vi "Resize Front Panel Main.vi"(0 "Left Listbox":refnum<vi>, 1 "Top Level VI":refnum<vi>, 2 "Stop":refnum<vi>, 3 "Number of Columns":i32=4, 5 "Right Listbox":refnum<vi>, 7 "Left Splitter":refnum<vi>, 9 "Right Splitter":refnum<vi>, 11 "error in (no error)":errorcluster, 12 "Left Pane Items":refnum<vi>[](array[refnum]), 13 "Mid Pane Items":refnum<vi>[](array[refnum]), 14 "Right Pane Items":refnum<vi>[](array[refnum])) -> (15 "error out":errorcluster)   [LabVIEW 2013]
uses:
  <vilib>/Utility/miscctls.llb/LVRectTypeDef.ctl
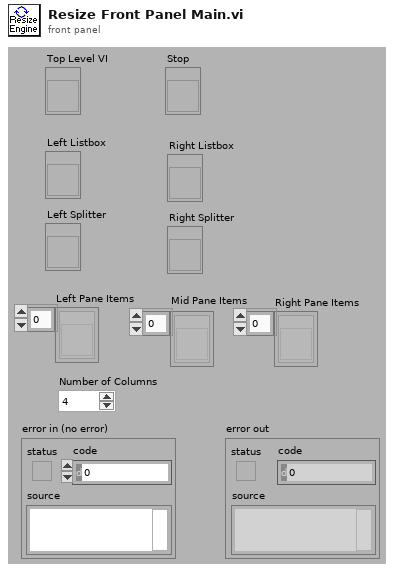
[diagram p1: front panel]
types:
  T1 = typedef "LVRectTypeDef.ctl" = cluster{"Left":i16, "Top":i16, "Right":i16, "Bottom":i16}
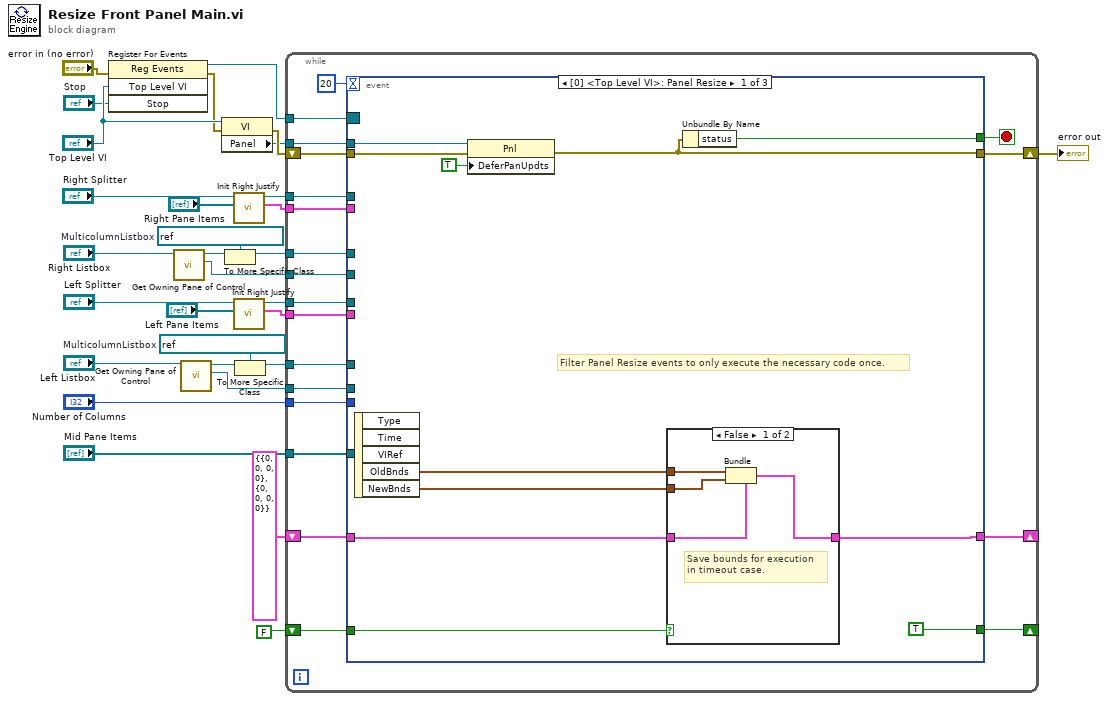
[diagram p0: block diagram]
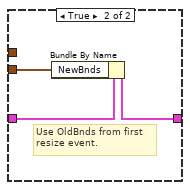
[diagram p2: hidden frame]
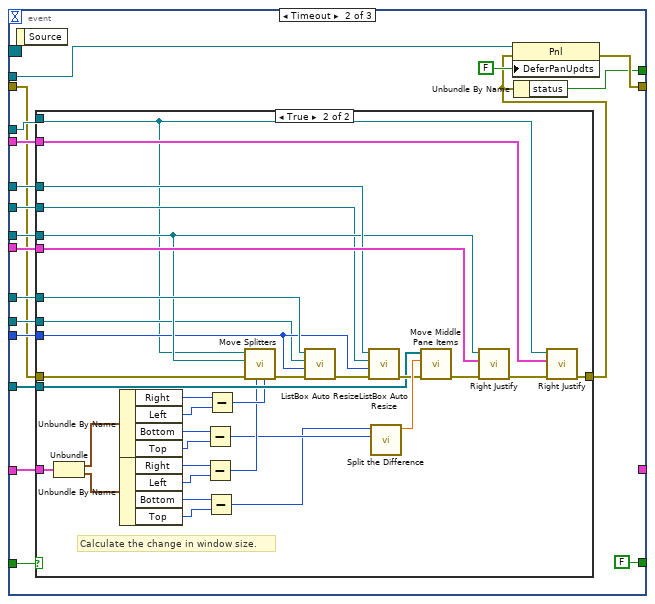
[diagram p3: hidden frame]
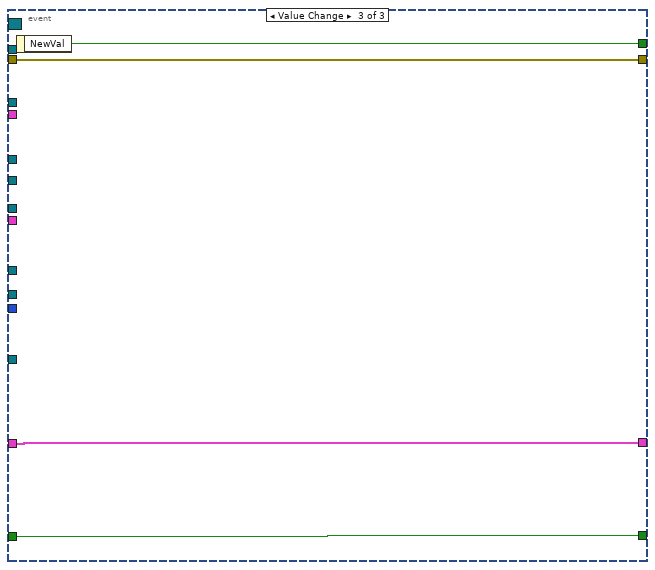
[diagram p5: hidden frame]
diagram:
  w7 = refnum<vi> refnum  # MulticolumnListbox
  w11 = refnum<vi> refnum  # MulticolumnListbox
  n1 = register-events(error in="error in (no error)", "Top Level VI", "Stop") -> (reference out=w22:refnum<event-registration>, error out=w21:errorcluster)  [unwired: 1 in]
  n2 = call "Get Owning Pane of Control.vi"("Ctl Refnum"="Right Listbox") -> ("Owning Pane"=w6:refnum<vi>, "dup Ctl Refnum"=w10:refnum<vi>)  [unwired: 8 in, 1 out]
  n3 = call "Get Owning Pane of Control.vi"("Ctl Refnum"="Left Listbox") -> ("Owning Pane"=w14:refnum<vi>, "dup Ctl Refnum"=w13:refnum<vi>)  [unwired: 8 in, 1 out]
  n4 = property class="VI"(reference="Top Level VI", error in=w21) -> (error out=w20:errorcluster, "Panel"=w5:refnum<vi>)  [unwired: 1 out]
  n5 = To More Specific Class(target class=w7, reference=w10) -> (specific class reference=w8:refnum<vi>)  [unwired: 1 in, 1 out]
  n6 = call "Init Right Justify.vi"("Right Justified Items"="Right Pane Items", "Splitter Reference"="Right Splitter") -> ("Position Coordinates"=w29:cluster{refnum<vi>, i32}[], "Splitter Reference"=w28:refnum<vi>)  [unwired: 7 in, 1 out]
  n7 = call "Init Right Justify.vi"("Right Justified Items"="Left Pane Items", "Splitter Reference"="Left Splitter") -> ("Position Coordinates"=w25:cluster{refnum<vi>, i32}[], "Splitter Reference"=w27:refnum<vi>)  [unwired: 7 in, 1 out]
  n8 = To More Specific Class(target class=w11, reference=w13) -> (specific class reference=w12:refnum<vi>)  [unwired: 1 in, 1 out]
  n9 = while {
    tunnel: w5 -> [w49]
    tunnel: w25 -> [w47]
    tunnel: w27 -> [w46]
    tunnel: w28 -> [w45]
    tunnel: w29 -> [w44]
    tunnel: w22 -> [w43]
    tunnel: w8 -> [w42]
    tunnel: w12 -> [w41]
    shift-right: [w39] -> w16
    shift-left: w20 -> [w40]
    tunnel: "Number of Columns" -> [w38]
    tunnel: "Mid Pane Items" -> [w37]
    tunnel: w14 -> [w36]
    tunnel: w6 -> [w35]
    shift-right: [w34] -> _
    shift-left: cluster{"OldBnds":T1, "NewBnds":T1} {"OldBnds"={"Left"=0, "Top"=0, "Right"=0, "Bottom"=0}, "NewBnds"={"Left"=0, "Top"=0, "Right"=0, "Bottom"=0}} -> [w33]
    shift-right: [w32] -> _
    shift-left: FALSE -> [w31]
    stop <- w50 stop-if-true
    n10 = event shown="[0] <Top Level VI>: Panel Resize" {
      selector: w43 -> [_ _ _]
      dyn-events: _ -> [_ _ _]
      timeout: 20 -> [_ _ _]
      tunnel: [w57 w69 w125] -> w50
      tunnel: w49 -> [w61 w71 _]
      tunnel: w47 -> [_ w87 _]
      tunnel: w46 -> [_ w84 _]
      tunnel: w45 -> [_ w78 _]
      tunnel: w44 -> [_ w79 _]
      tunnel: w42 -> [_ w86 _]
      tunnel: w41 -> [_ w85 _]
      tunnel: w40 -> [w59 w73 w124]
      tunnel: [w58 w72 w124] -> w39
      tunnel: w38 -> [_ w82 _]
      tunnel: w37 -> [_ w83 _]
      tunnel: w36 -> [_ w81 _]
      tunnel: w35 -> [_ w80 _]
      tunnel: [w51 _ w123] -> w34
      tunnel: w33 -> [w52 w77 w123]
      tunnel: [TRUE FALSE w122] -> w32
      tunnel: w31 -> [w55 w75 w122]
      event Panel Resize {
        # "Filter Panel Resize events to only execute the necessary code once."
        n11 = event-data() -> ("OldBnds"=w54:T1, "NewBnds"=w53:T1)  [unwired: 1 in, 3 out]
        n12 = property class="Pnl"(reference=w61, error in=w59, "DeferPanUpdts"=TRUE ("Defer Panel Updates")) -> (error out=w58:errorcluster)  [unwired: 1 out]
        n13 = case shown="False" w55 {
          tunnel: w54 -> [w65 _]
          tunnel: w53 -> [w64 w66]
          tunnel: w52 -> [w63 w68]
          tunnel: [w62 w67] -> w51
          frame False {
            # "Save bounds for execution\nin timeout case."
            n14 = Bundle(cluster=w63, "OldBnds"=w65, "NewBnds"=w64) -> (w62:cluster{"OldBnds":T1, "NewBnds":T1})
          }
          frame True {
            # "Use OldBnds from first\nresize event."
            n15 = Bundle By Name(cluster=w68, "NewBnds"=w66) -> (w67:cluster{"OldBnds":T1, "NewBnds":T1})
          }
        }
        n16 = Unbundle By Name(w58) -> ("status"=w57:bool)
      }
      event Timeout {
        n17 = event-data() -> ()  [unwired: 1 in, 1 out]
        n18 = case shown="True" w75 {
          tunnel: w87 -> [_ w117]
          tunnel: w86 -> [_ w116]
          tunnel: w85 -> [_ w115]
          tunnel: w84 -> [_ w114]
          tunnel: w83 -> [_ w113]
          tunnel: w82 -> [_ w112]
          tunnel: w81 -> [_ w111]
          tunnel: w80 -> [_ w110]
          tunnel: [w88 w108] -> w70
          tunnel: w79 -> [_ w106]
          tunnel: w73 -> [w88 w105]
          tunnel: w78 -> [_ w92]
          tunnel: w77 -> [_ w91]
          frame False {
          }
          frame True {
            # "Calculate the change in window size."
            n19 = Unbundle(w91) -> ("OldBnds"=w90:T1, "NewBnds"=w89:T1)
            n20 = Unbundle By Name(w90) -> ("Right"=w103:i16, "Left"=w104:i16, "Bottom"=w98:i16, "Top"=w97:i16)
            n21 = Unbundle By Name(w89) -> ("Right"=w101:i16, "Left"=w100:i16, "Bottom"=w95:i16, "Top"=w94:i16)
            n22 = Subtract(x=w98, y=w97) -> (x-y=w96:i16)
            n23 = Subtract(x=w101, y=w100) -> (x-y=w99:i16)
            n24 = Subtract(x=w95, y=w94) -> (x-y=w93:i16)
            n25 = Subtract(x=w103, y=w104) -> (x-y=w102:i16)
            n26 = call "Move Splitters.vi"("Old Width"=w102, "New Width"=w99, "error in"=w105, "Left Splitter"=w114, "Right Splitter"=w92) -> ("error out"=w120:errorcluster)  [unwired: 6 in]
            n27 = call "ListBox Auto Resize.vi"("error in (no error)"=w120, "Number of Columns"=w112, "Owning Pane"=w111, "MultiColumn Listbox"=w115) -> ("error out"=w121:errorcluster)  [unwired: 7 in]
            n28 = call "ListBox Auto Resize.vi"("error in (no error)"=w121, "Number of Columns"=w112, "Owning Pane"=w110, "MultiColumn Listbox"=w116) -> ("error out"=w118:errorcluster)  [unwired: 7 in]
            n29 = call "Split the Difference.vi"("Y"=w96, "X"=w93) -> ("Half the Difference"=w119:dbl)  [unwired: 9 in]
            n30 = call "Move Middle Pane Items.vi"("error in"=w118, "Vertical Distance to Move"=w119, "Object References"=w113) -> ("error out"=w109:errorcluster)  [unwired: 8 in]
            n31 = call "Right Justify.vi"("error in"=w109, "Position Coordinates"=w117, "Splitter Reference"=w114) -> ("error out"=w107:errorcluster)  [unwired: 8 in]
            n32 = call "Right Justify.vi"("error in"=w107, "Position Coordinates"=w106, "Splitter Reference"=w92) -> ("error out"=w108:errorcluster)  [unwired: 8 in]
          }
        }
        n33 = property class="Pnl"(reference=w71, error in=w70, "DeferPanUpdts"=FALSE ("Defer Panel Updates")) -> (error out=w72:errorcluster)  [unwired: 1 out]
        n34 = Unbundle By Name(w70) -> ("status"=w69:bool)
      }
      event Value Change {
        n35 = event-data() -> ("NewVal"=w125:bool)  [unwired: 1 in]
      }
    }
  }
  "error out" <- w16
